vi "Write delimiter.vi"(8 "error in (no error)":errorcluster, 10 "delimiter":string=",", 11 "CSVLayout in":refnum<class "CSVLayout.lvclass">) -> (0 "error out":errorcluster, 3 "CSVLayout out":refnum<class "CSVLayout.lvclass">)   [LabVIEW 2026, in "Lumberjack.lvlib" / "CSVLayout.lvclass"]
doc: "Stores the single-character column delimiter into the layout's private data.\nClass private-data accessor; sets the `delimiter` field (e.g. \",\" for CSV or a tab for TSV). No side effects.\nLumberjack.lvlib, CSVLayout.lvclass, public."
uses:
  CSVLayout.lvclass
  CSVLayout.lvclass/CSVLayout.ctl
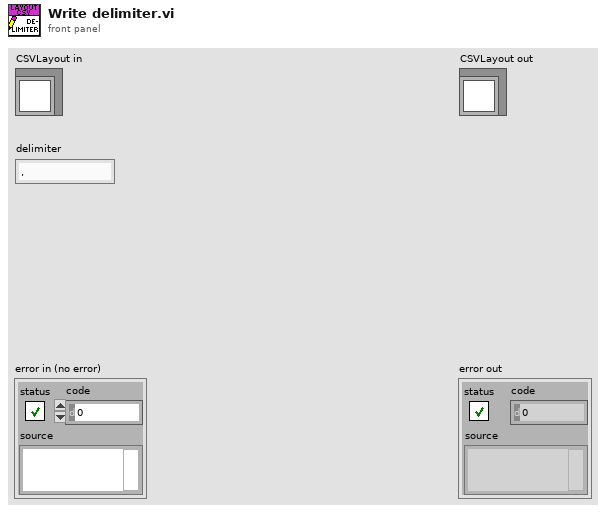
[diagram p1: front panel]
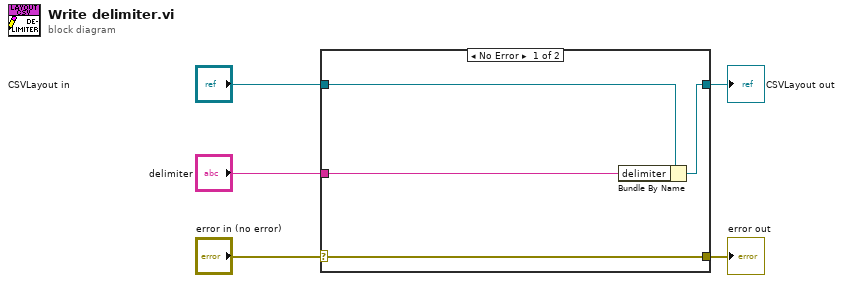
[diagram p0: block diagram]
diagram:
  n1 = case shown="No Error" "error in (no error)" {
    selector: "error in (no error)" -> [w9 w10]
    tunnel: [w9 w10] -> w4
    tunnel: [w7 w11] -> w2
    tunnel: "CSVLayout in" -> [w8 w11]
    tunnel: "delimiter" -> [w6 _]
    frame No Error {
      n2 = Bundle By Name(cluster=w8, "delimiter"=w6) -> (w7:refnum<class "CSVLayout.lvclass">)
    }
    frame Error {
    }
  }
  "error out" <- w4
  "CSVLayout out" <- w2
